vi "Generate_WayPoints_Hopping_multipleCV_Surface.vi"(11 "Input Cluster":T2={"Scan Rate (um/s)"=15.0, "X Start"=15.0, "X End"=15.0, "Y Start"=15.0, "Y End"=15.0, " Z Start"=15.0, "HoppingDistance"=1.0, "V"=15.0, "Z End"=15.0, "Approach Rate Hopping (um/s)"=15.0, "Retrack Rate (um/s)"=15.0, "V 2"=15.0, "Approach Rate (um/s)"=15.0, "V 3"=15.0, "CV Rate / V/s"=15.0, "V 4"=15.0, "V 1"=15.0, "HoldTime1/s"=15.0, "Hold time 2 / s"=15.0, "Hold time 3/ s"=15.0, "No. of Cycles"=15}) -> (0 "output cluster":T1)   [LabVIEW 2023]
uses:
  TypeDefs/WayPointCluster.ctl
  TypeDefsControls/Time.ctl
  User_Vi/Settings.vi
panel:
  in  "WayPointCluster":T1
  out "Y  P":dbl
  out "X  P":dbl
  out "HoppingDistanceX":dbl
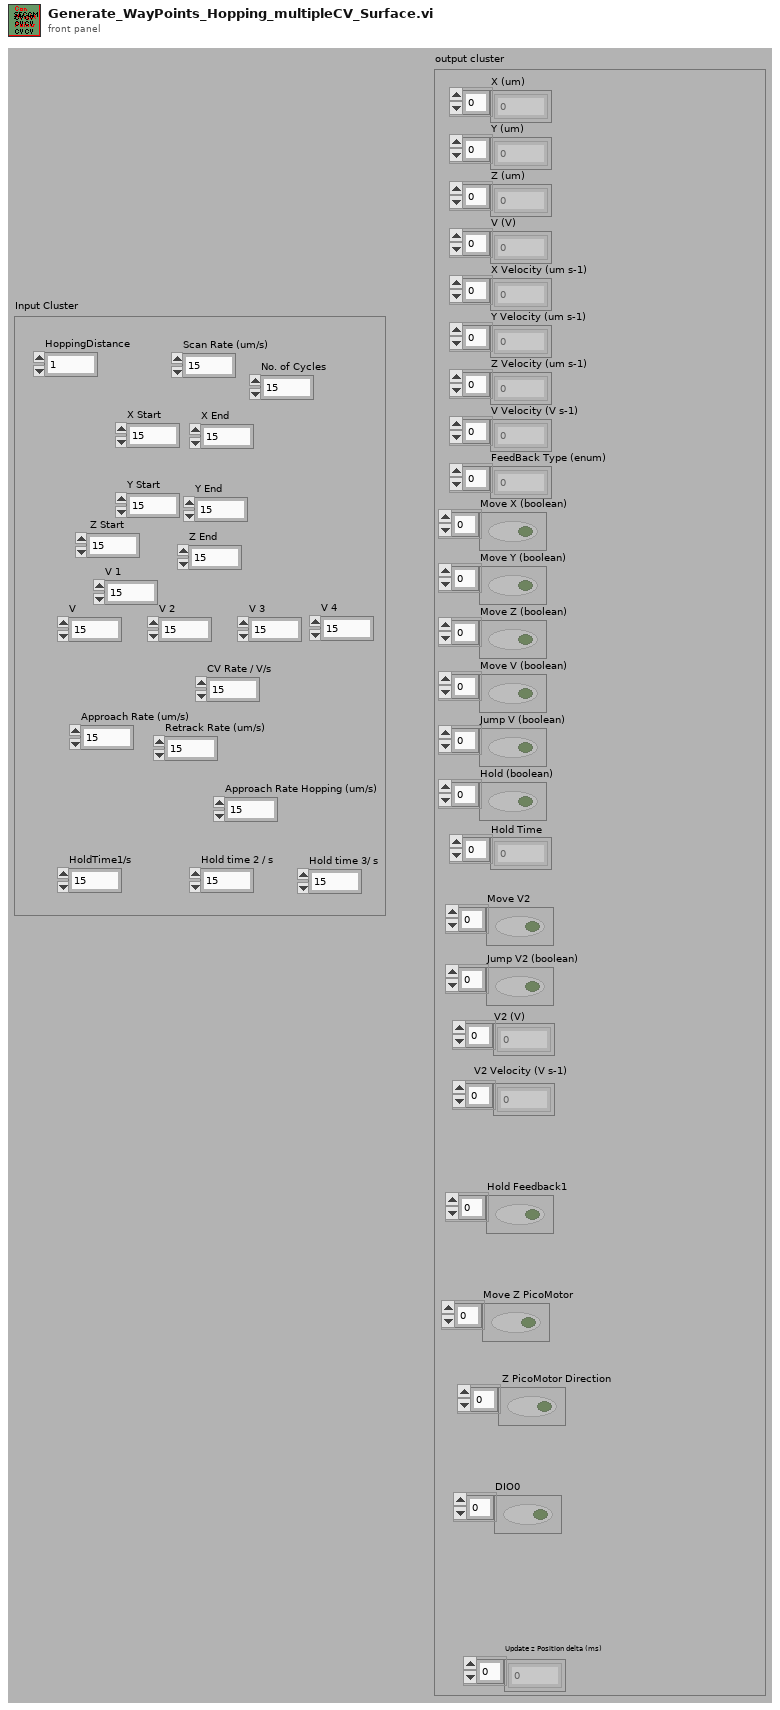
[diagram p1: front panel]
types:
  T1 = typedef "WayPointCluster.ctl" = cluster{"X (um)":dbl[], "Y (um)":dbl[], "Z (um)":dbl[], "V (V)":dbl[], "X Velocity (um s-1)":dbl[], "Y Velocity (um s-1)":dbl[], "Z Velocity (um s-1)":dbl[], "V Velocity (V s-1)":dbl[], "FeedBack Type (enum)":u16[], "Move X (boolean)":bool[], "Move Y (boolean)":bool[], "Move Z (boolean)":bool[], "Move V (boolean)":bool[], "Jump V (boolean)":bool[], "Hold (boolean)":bool[], "Hold Time":u32[], "V2 (V)":dbl[], "Move V2":bool[], "V2 Velocity (V s-1)":dbl[], "Jump V2 (boolean)":bool[], "Update z Position delta (ms)":i16[], "Hold Feedback1":bool[], "Move Z PicoMotor":bool[], " Z PicoMotor Direction":bool[], "DIO0":bool[]}
  T2 = cluster{"Scan Rate (um/s)":dbl, "X Start":dbl, "X End":dbl, "Y Start":dbl, "Y End":dbl, " Z Start":dbl, "HoppingDistance":dbl, "V":dbl, "Z End":dbl, "Approach Rate Hopping (um/s)":dbl, "Retrack Rate (um/s)":dbl, "V 2":dbl, "Approach Rate (um/s)":dbl, "V 3":dbl, "CV Rate / V/s":dbl, "V 4":dbl, "V 1":dbl, "HoldTime1/s":dbl, "Hold time 2 / s":dbl, "Hold time 3/ s":dbl, "No. of Cycles":i32}
  T3 = typedef "Time.ctl" = dbl
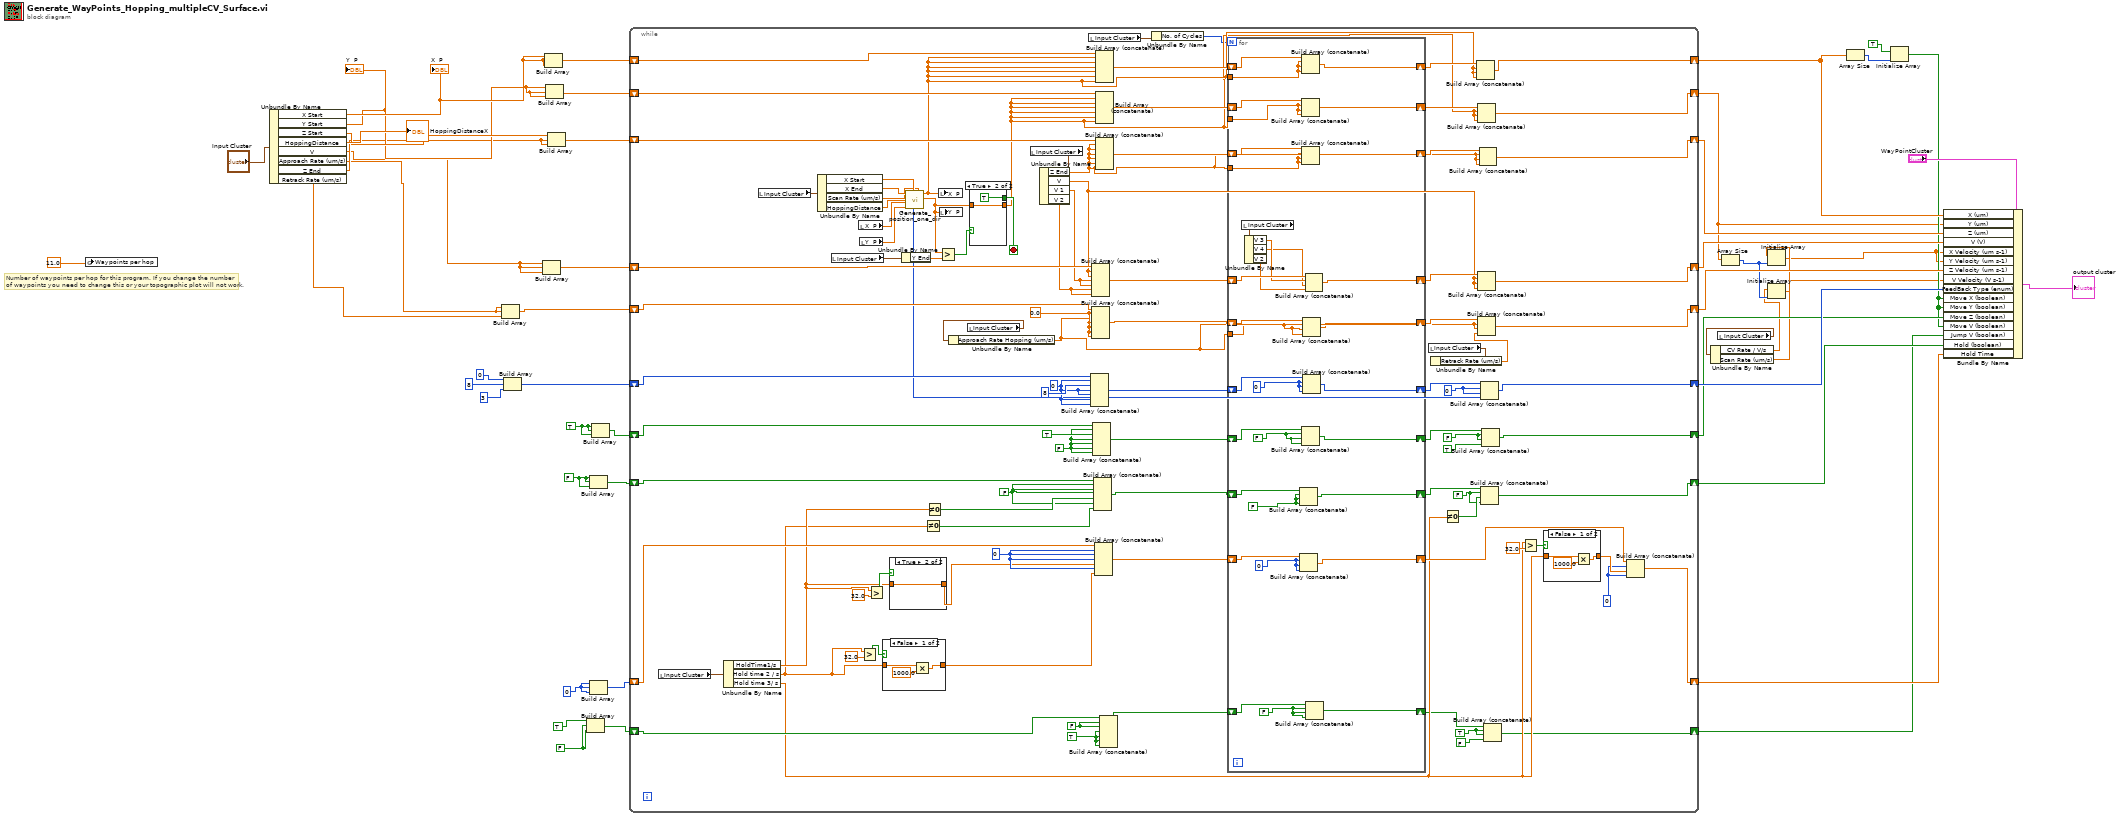
[diagram p0: block diagram]
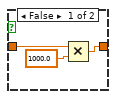
[diagram p3: hidden frame]
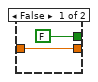
[diagram p5: hidden frame]
diagram:
  w23 = FALSE
  w2 = FALSE
  w24 = u32 0 ("element")
  w21 = TRUE
  # "Number of waypoints per hop for this program. If you change the number\nof waypoints you need to change this or your topographic plot will not work."
  n1 = global write "Settings.vi" "Waypoints per hop"(11.0) -> ()
  n2 = Unbundle By Name("Input Cluster") -> ("X Start"=w36:dbl, "Y Start"=w35:dbl, "Z Start"=w37:dbl, "HoppingDistance"=→"HoppingDistanceX":dbl, "V"=w33:dbl, "Approach Rate (um/s)"=w20:dbl, "Z End"=w34:dbl, "Retrack Rate (um/s)"=w32:dbl)
  "X  P" <- w36
  "Y  P" <- w35
  n3 = Build Array(w20, w20, w32) -> (w42:dbl[])
  n4 = Build Array(u16 0 ("element"), u16 8, u16 3 ("element")) -> (w40:u16[])
  n5 = Build Array(w33, w33, w33) -> (w44:dbl[])
  n6 = Build Array(w36, w36, w36) -> (w48:dbl[])
  n7 = Build Array(w35, w35, w35) -> (w47:dbl[])
  n8 = Build Array(w37, w34, w34) -> (w46:dbl[])
  n9 = Build Array(TRUE, w2, w2) -> (w27:bool[])
  n10 = Build Array(w23, w23, w23) -> (w22:bool[])
  n11 = Build Array(w24, w24, w24) -> (w30:u32[])
  n12 = Build Array(w21, w21, w21) -> (w17:bool[])
  n13 = while {
    shift-right: [w59] -> w13
    shift-left: w48 -> [w139]
    shift-right: [w58] -> w8
    shift-left: w47 -> [w138]
    shift-right: [w57] -> w45
    shift-left: w46 -> [w137]
    shift-right: [w56] -> w43
    shift-left: w44 -> [w136]
    shift-right: [w55] -> w41
    shift-left: w42 -> [w135]
    shift-right: [w54] -> w39
    shift-left: w40 -> [w146]
    shift-right: [w53] -> w14
    shift-left: w17 -> [w134]
    shift-right: [w52] -> w29
    shift-left: w22 -> [w132]
    shift-right: [w63] -> w28
    shift-left: w30 -> [w131]
    shift-right: [w51] -> w26
    shift-left: w27 -> [w128]
    stop <- w141 stop-if-true
    w61 = TRUE
    w65 = u32 0 ("element")
    w68 = FALSE
    w72 = FALSE
    w75 = u16 0 ("element")
    w106 = TRUE
    w127 = FALSE
    w129 = u32 0 ("element")
    w105 = FALSE
    w126 = FALSE
    w102 = 0.0 ("element")
    w101 = u16 0 ("element")
    n14 = local read "Input Cluster"() -> (w130:T2)
    n15 = Unbundle By Name(w130) -> ("HoldTime1/s"=w109:dbl, "Hold time 2 / s"=w107:dbl, "Hold time 3/ s"=w64:dbl)
    n16 = local read "Input Cluster"() -> (w147:T2)
    n17 = Unbundle By Name(w147) -> ("X Start"=w123:dbl, "X End"=w122:dbl, "Scan Rate (um/s)"=w121:dbl, "HoppingDistance"=w120:dbl)
    n18 = local read "Input Cluster"() -> (w144:T2)
    n19 = local read "X  P"() -> (w125:dbl)
    n20 = local read "Y  P"() -> (w124:dbl)
    n21 = Greater?(x=w107, y=T3 32.0) -> (0:w116:bool)
    n22 = Greater?(x=w109, y=T3 32.0) -> (0:w114:bool)
    n23 = case shown="False" w116 {
      tunnel: w107 -> [w191 w192]
      tunnel: [w190 w192] -> w110
      frame False {
        n24 = Multiply(x=w191, y=1000.0) -> (x*y=w190:dbl)
      }
      frame True {
      }
    }
    n25 = case shown="True" w114 {
      tunnel: w109 -> [w187 w188]
      tunnel: [w186 w188] -> w111
      frame False {
        n26 = Multiply(x=w187, y=1000.0) -> (x*y=w186:dbl)
      }
      frame True {
      }
    }
    n27 = Unbundle By Name(w144) -> ("Y End"=w143:dbl)
    n28 = call "Generate_position_one_dir.vi"("HoppingDistance input"=w120, "X Start input"=w123, "Y P input"=w124, "X P input"=w125, "Scan Rate (um/s) input"=w121, "X end input"=w122) -> ("Y P output"=w119:dbl, "X P output"=w87:dbl, "Feedback type retraction output"=w74:u64)  [unwired: 1 in, 2 out]
    n29 = Not Equal To 0?(x=w107) -> (x != 0?=w100:bool)
    n30 = Not Equal To 0?(x=w109) -> (x != 0?=w108:bool)
    n31 = local write "X  P"(w87) -> ()
    n32 = local write "Y  P"(w119) -> ()
    n33 = Greater?(x=w119, y=w143) -> (0:w142:bool)
    n34 = local read "Input Cluster"() -> (w140:T2)
    n35 = Unbundle By Name(w140) -> ("Approach Rate Hopping (um/s)"=w78:dbl)
    n36 = case shown="True" w142 {
      tunnel: w119 -> [w194 w196]
      tunnel: [w194 w196] -> w85
      tunnel: [FALSE TRUE] -> w141
      frame False {
      }
      frame True {
      }
    }
    n37 = local read "Input Cluster"() -> (w145:T2)
    n38 = Unbundle By Name(w145) -> ("Z End"=w83:dbl, "V"=w81:dbl, "V 1"=w104:dbl, "V 2"=w103:dbl)
    n39 = local read "Input Cluster"() -> (w99:T2)
    n40 = Build Array (concatenate)(w146, w101, u16 8, w101, w101, w101, w101) -> (w93:u64[])
    n41 = Build Array (concatenate)(w136, w81, w81, w104, w104, w103, w103) -> (w95:dbl[])
    n42 = Build Array (concatenate)(w135, w102, w78, w102, w102, w102, w102) -> (w94:dbl[])
    n43 = Build Array (concatenate)(w134, w126, TRUE, w126, w126, w126, w126) -> (w92:bool[])
    n44 = Build Array (concatenate)(w132, w105, w105, w105, w108, w105, w100) -> (w91:bool[])
    n45 = Build Array (concatenate)(w131, w129, w129, w129, w111, w129, w110) -> (w90:dbl[])
    n46 = Build Array (concatenate)(w137, w83, w83, w83, w83, w83, w83) -> (w96:dbl[])
    n47 = Build Array (concatenate)(w139, w87, w87, w87, w87, w87, w87) -> (w98:dbl[])
    n48 = Build Array (concatenate)(w138, w85, w85, w85, w85, w85, w85) -> (w97:dbl[])
    n49 = Build Array (concatenate)(w128, w127, w127, w106, w106, w106, w106) -> (w89:bool[])
    n50 = Unbundle By Name(w99) -> ("No. of Cycles"=w50:i32)
    n51 = for {
      N: w50 -> [_]
      shift-right: [w179] -> w88
      shift-left: w98 -> [w180]
      shift-right: [w175] -> w86
      shift-left: w97 -> [w177]
      shift-right: [w172] -> w84
      shift-left: w96 -> [w174]
      shift-right: [w166] -> w82
      shift-left: w95 -> [w170]
      shift-right: [w163] -> w80
      shift-left: w94 -> [w165]
      shift-right: [w160] -> w76
      shift-left: w93 -> [w162]
      shift-right: [w154] -> w73
      shift-left: w92 -> [w159]
      shift-right: [w155] -> w69
      shift-left: w91 -> [w157]
      shift-right: [w151] -> w67
      shift-left: w90 -> [w153]
      shift-right: [w148] -> w62
      shift-left: w89 -> [w150]
      tunnel: w87 -> [w178]
      tunnel: w85 -> [w176]
      tunnel: w83 -> [w173]
      tunnel: w78 -> [w164]
      w149 = FALSE
      w152 = u32 0 ("element")
      w156 = FALSE
      w158 = FALSE
      w161 = u16 0 ("element")
      n52 = local read "Input Cluster"() -> (w171:T2)
      n53 = Unbundle By Name(w171) -> ("V 3"=w169:dbl, "V 4"=w168:dbl, "V 2"=w167:dbl)
      n54 = Build Array (concatenate)(w157, w156, w156, w156) -> (w155:bool[])
      n55 = Build Array (concatenate)(w153, w152, w152, w152) -> (w151:dbl[])
      n56 = Build Array (concatenate)(w180, w178, w178, w178) -> (w179:dbl[])
      n57 = Build Array (concatenate)(w177, w176, w176, w176) -> (w175:dbl[])
      n58 = Build Array (concatenate)(w174, w173, w173, w173) -> (w172:dbl[])
      n59 = Build Array (concatenate)(w159, w158, w158, w158) -> (w154:bool[])
      n60 = Build Array (concatenate)(w162, w161, w161, w161) -> (w160:u64[])
      n61 = Build Array (concatenate)(w165, w164, w164, w164) -> (w163:dbl[])
      n62 = Build Array (concatenate)(w170, w169, w168, w167) -> (w166:dbl[])
      n63 = Build Array (concatenate)(w150, w149, w149, w149) -> (w148:bool[])
    }
    n64 = local read "Input Cluster"() -> (w79:T2)
    n65 = Unbundle By Name(w79) -> ("Retrack Rate (um/s)"=w77:dbl)
    n66 = Not Equal To 0?(x=w64) -> (x != 0?=w70:bool)
    n67 = Build Array (concatenate)(w88, w87, w87, w87) -> (w59:dbl[])
    n68 = Build Array (concatenate)(w86, w85, w85, w85) -> (w58:dbl[])
    n69 = Build Array (concatenate)(w82, w81, w81, w81) -> (w56:dbl[])
    n70 = Build Array (concatenate)(w80, w78, w78, w77) -> (w55:dbl[])
    n71 = Build Array (concatenate)(w84, w83, w83, w83) -> (w57:dbl[])
    n72 = Build Array (concatenate)(w76, w75, w75, w74) -> (w54:u64[])
    n73 = Build Array (concatenate)(w69, w68, w70, w68) -> (w52:bool[])
    n74 = Build Array (concatenate)(w73, w72, w72, TRUE) -> (w53:bool[])
    n75 = Build Array (concatenate)(w62, w61, w61, FALSE) -> (w51:bool[])
    n76 = Greater?(x=w64, y=T3 32.0) -> (0:w112:bool)
    n77 = case shown="False" w112 {
      tunnel: [w183 w184] -> w66
      tunnel: w64 -> [w181 w184]
      frame False {
        n78 = Multiply(x=w181, y=1000.0) -> (x*y=w183:dbl)
      }
      frame True {
      }
    }
    n79 = Build Array (concatenate)(w67, w65, w66, w65) -> (w63:dbl[])
  }
  n80 = local read "Input Cluster"() -> (w9:T2)
  n81 = Unbundle By Name(w9) -> ("CV Rate / V/s"=w6:dbl, "Scan Rate (um/s)"=w5:dbl)
  n82 = Array Size(array=w8) -> (size(s)=w7:i32)
  n83 = Initialize Array(w5, w7) -> (w4:dbl[])
  n84 = Initialize Array(w6, w7) -> (w3:dbl[])
  n85 = Array Size(array=w13) -> (size(s)=w12:i32)
  n86 = Initialize Array(TRUE, w12) -> (w10:bool[])
  n87 = Bundle By Name(cluster="WayPointCluster", "X (um)"=w13, "Y (um)"=w8, "Z (um)"=w45, "V (V)"=w43, "X Velocity (um s-1)"=w4, "Y Velocity (um s-1)"=w4, "Z Velocity (um s-1)"=w41, "V Velocity (V s-1)"=w3, "FeedBack Type (enum)"=w39, "Move X (boolean)"=w10, "Move Y (boolean)"=w10, "Move Z (boolean)"=w14, "Move V (boolean)"=w10, "Jump V (boolean)"=w26, "Hold (boolean)"=w29, "Hold Time"=w28) -> (→"output cluster":T1)
